vi "load firmware.vi"(7 "board_num":u16, 8 "error in (no error)":errorcluster, 9 "filename":string, 10 "store":bool, 11 "identifier":string) -> (0 "error out":errorcluster, 1 "filename out":string, 3 "function return":u32)   [LabVIEW 2015, in "XGL_DPP.lvlib"]
doc: "EXTERN DECLSPEC uint32_t CALL_CONV load_firmware(const char * identifier, bool store, char * filename, uint16_t board_num );"
uses:
  XGL_DPP.lvlib
  XGL_DPP.dll
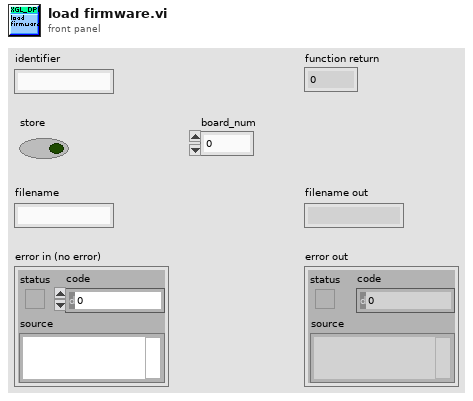
[diagram p1: front panel]
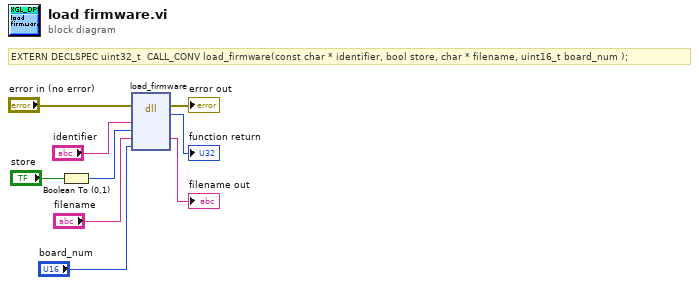
[diagram p0: block diagram]
diagram:
  # "EXTERN DECLSPEC uint32_t  CALL_CONV load_firmware(const char * identifier, bool store, char * filename, uint16_t board_num );"
  n1 = Boolean To (0,1)(Boolean="store") -> (0, 1=w6:i16)
  n2 = dll-call lib="D:/Users/XRF/Desktop/Scanning Software_Demokritos_2015_v7/libs/Vis_2/XGL_DPP.*" fn="load_firmware"(error in="error in (no error)", "identifier"="identifier", "store"=w6, "filename"="filename", "board_num"="board_num") -> (error out=→"error out":errorcluster, →"function return":u32, "filename"=→"filename out":string)  [unwired: 5 in, 1 out]
